vi "Task5.vi"() -> ()   [LabVIEW 2017]
panel:
  out "Numeric":u8
  in  "8bit switches":bool[](array[boolean])
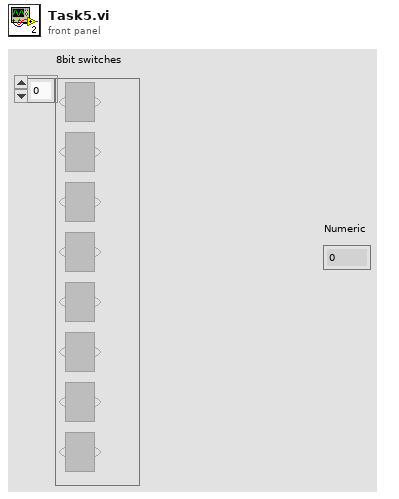
[diagram p1: front panel]
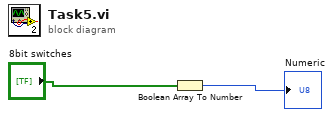
[diagram p0: block diagram]
diagram:
  n1 = Boolean Array To Number(Boolean array="8bit switches") -> (number=→"Numeric":u32)
